vi "RT - Sender.vi"() -> ()   [LabVIEW 2017]
panel:
  in  "stop":bool
  out "String":string
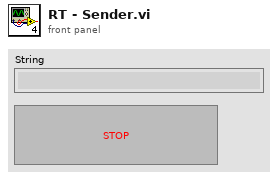
[diagram p1: front panel]
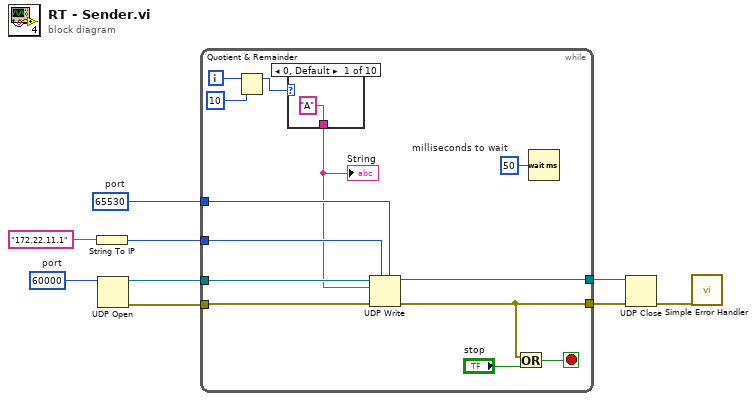
[diagram p0: block diagram]
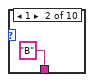
[diagram p2: hidden frame]
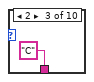
[diagram p3: hidden frame]
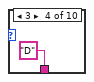
[diagram p4: hidden frame]
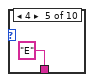
[diagram p5: hidden frame]
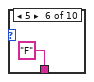
[diagram p6: hidden frame]
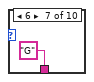
[diagram p7: hidden frame]
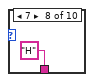
[diagram p8: hidden frame]
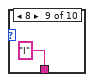
[diagram p9: hidden frame]
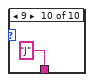
[diagram p10: hidden frame]
diagram:
  w4 = u16 65530  # port
  w9 = u16 60000  # port
  n1 = String To IP(1:"172.22.11.1") -> (0:w5:u32)
  n2 = UDP Open(11:w9) -> (port=w7:refnum<k16>, 0:w8:errorcluster)  [unwired: 4 in, 1 out]
  n3 = while {
    tunnel: w8 -> [w20]
    tunnel: w7 -> [w21]
    tunnel: w5 -> [w19]
    tunnel: w4 -> [w18]
    tunnel: [w17] -> w3
    tunnel: [w15] -> w2
    i -> [w13]
    stop <- w16 stop-if-true
    w22 = u32 50  # milliseconds to wait
    n4 = Quotient & Remainder(x=w13, y=10) -> (x-y*floor(x/y)=w11:i32)  [unwired: 1 out]
    n5 = case shown="0, Default" w11 {
      tunnel: ["A" "B" "C" "D" "E" "F" "G" "H" "I" "J"] -> w10
      frame 0, Default {
      }
      frame 1 {
      }
      frame 2 {
      }
      frame 3 {
      }
      frame 4 {
      }
      frame 5 {
      }
      frame 6 {
      }
      frame 7 {
      }
      frame 8 {
      }
      frame 9 {
      }
    }
    "String" <- w10
    n6 = UDP Write(address=w19, port or service name=w18, connection ID=w21, data in=w10, 8:w20) -> (error out=w15:errorcluster, 3:w17:refnum<k16>)  [unwired: 1 in]
    n7 = Or(x=w15, y="stop") -> (x .or. y?=w16:bool)
    n8 = Wait (ms)(milliseconds to wait=w22) -> ()  [unwired: 1 out]
  }
  n9 = UDP Close(connection ID=w3, 8:w2) -> (error out=w1:errorcluster)  [unwired: 1 out]
  n10 = call <vilib>:"Simple Error Handler.vi"("error in (no error)"=w1) -> ()  [unwired: 4 in, 5 out]
